vi "SET ALLIANCE.vi"(8 "error in (no error)":errorcluster, 11 "stack name":string="DB/Button 0") -> (0 "error out":errorcluster, 3 "Alliance":T1)   [LabVIEW 2023]
uses:
  <vilib>/Rock Robotics/WPI/DriverStation/WPI_DriverStationAllianceInfo.ctl
  <vilib>/Rock Robotics/Network Tables/NT Read Boolean.vi
  Global odometry.vi
  <vilib>/Rock Robotics/Network Tables/NT Write String.vi
  <vilib>/Rock Robotics/Network Tables/NT Write Boolean.vi
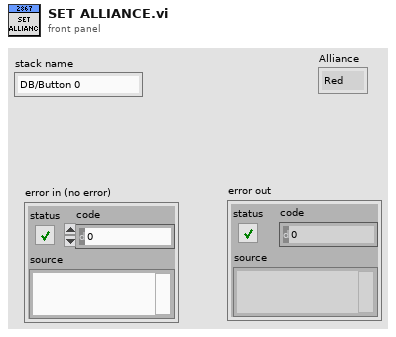
[diagram p1: front panel]
types:
  T1 = typedef "WPI_DriverStationAllianceInfo.ctl" = enum16{"Red", "Blue", "Invalid"}
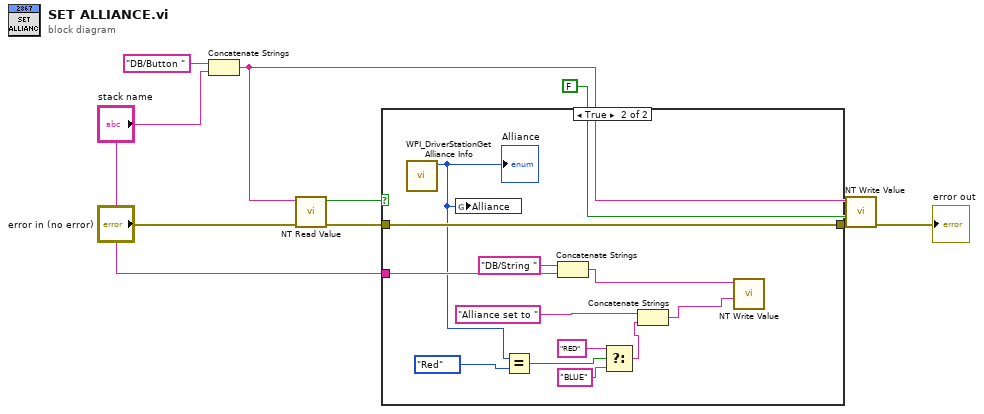
[diagram p0: block diagram]
diagram:
  n1 = Concatenate Strings("DB/Button " ("string"), "stack name") -> (w3:string)
  n2 = call-poly <vilib>:"NT Read Value.vi"("error in"="error in (no error)", "name"=w3) -> ("error out"=w5:errorcluster, "value"=w9:bool)  [unwired: 7 in, 1 out]
  n3 = case shown="True" w9 {
    tunnel: w5 -> [_ w21]
    tunnel: [_ w21] -> w4
    tunnel: "stack name" -> [_ w19]
    frame False {
    }
    frame True {
      n4 = call <vilib>:"WPI_DriverStationGet Alliance Info.vi"() -> ("Alliance"=w12:T1)  [unwired: 6 in, 5 out]
      "Alliance" <- w12
      n5 = global write "Global odometry.vi" "Alliance"(w12) -> ()
      n6 = Equal?(x=w12, y=WPI_DriverStationAllianceInfo."Red" ("Alliance 2")) -> (x = y?=w14:bool)
      n7 = Concatenate Strings("DB/String " ("string"), w19) -> (w18:string)
      n8 = Select(t="RED", s=w14, f="BLUE") -> (s? t:f=w11:string)
      n9 = Concatenate Strings("Alliance set to " ("string"), w11) -> (w10:string)
      n10 = call-poly <vilib>:"NT Write Value.vi"("value"=w10, "name"=w18) -> ()  [unwired: 9 in, 1 out]
    }
  }
  n11 = call-poly <vilib>:"NT Write Value.vi"("error in"=w4, "value"=FALSE, "name"=w3) -> ("error out"=→"error out":errorcluster)  [unwired: 8 in]
